vi "Update display current.vi"(8 "error in (no error)":errorcluster, 11 "StageSPIM in":refnum<class "StageSPIM.lvclass">) -> (0 "error out":errorcluster, 3 "StageSPIM out":refnum<class "StageSPIM.lvclass">)   [LabVIEW 2012, in "StageSPIM.lvclass"]
uses:
  StageSPIM.lvclass
  StageSPIM.lvclass/StageSPIM.ctl
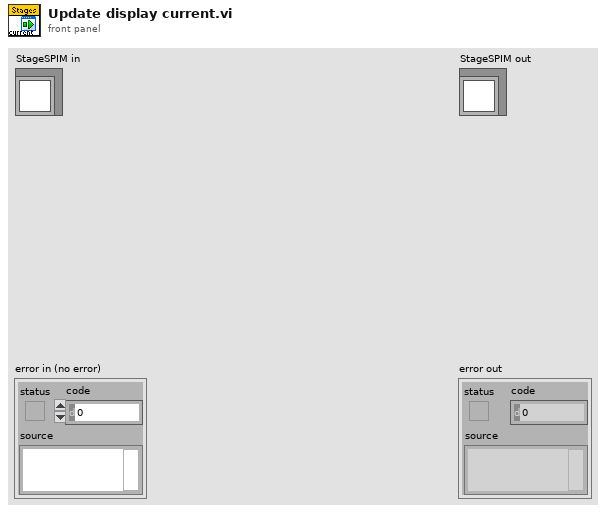
[diagram p1: front panel]
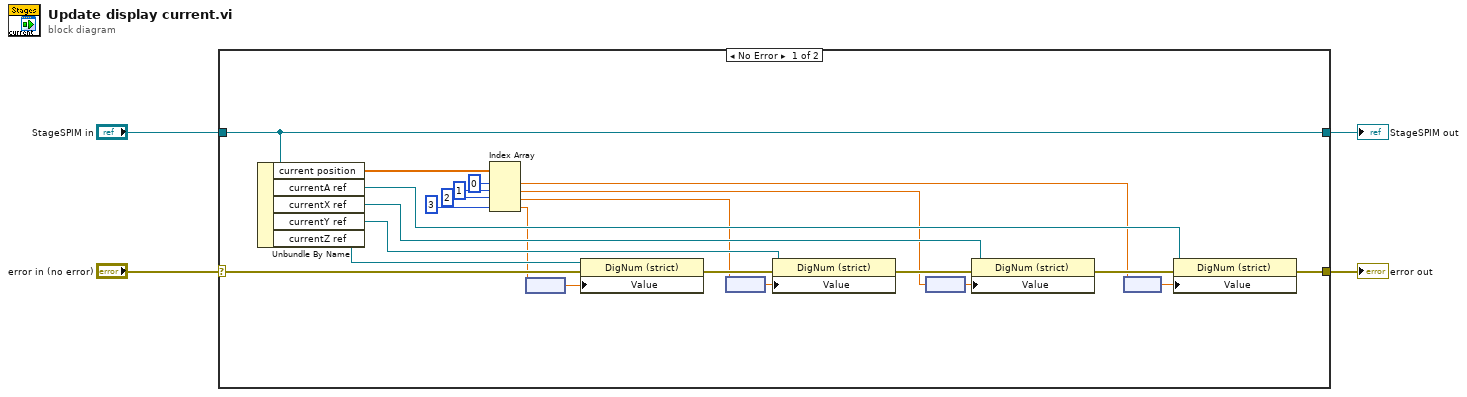
[diagram p0: block diagram]
diagram:
  n1 = case shown="No Error" "error in (no error)" {
    selector: "error in (no error)" -> [w21 w29]
    tunnel: [w13 w29] -> w3
    tunnel: [w27 w28] -> w1
    tunnel: "StageSPIM in" -> [w27 w28]
    frame No Error {
      n2 = Unbundle By Name(w27) -> ("current position"=w26:dbl[], "currentA ref"=w17:refnum<vi>, "currentX ref"=w18:refnum<vi>, "currentY ref"=w19:refnum<vi>, "currentZ ref"=w20:refnum<vi>)
      n3 = Index Array(array=w26, index #1=0 ("index"), index #2=1 ("index"), index #3=2 ("index"), index #4=3 ("index")) -> (element #1=w5:dbl, element #2=w7:dbl, element #3=w9:dbl, element #4=w11:dbl)
      n4 = node(w11) -> (w12:dbl[unit])
      n5 = property class="DigNum (strict)"(reference=w20, error in=w21, "Value"=w12) -> (error out=w16:errorcluster)  [unwired: 1 out]
      n6 = node(w9) -> (w10:dbl[unit])
      n7 = property class="DigNum (strict)"(reference=w19, error in=w16, "Value"=w10) -> (error out=w15:errorcluster)  [unwired: 1 out]
      n8 = node(w7) -> (w8:dbl[unit])
      n9 = property class="DigNum (strict)"(reference=w18, error in=w15, "Value"=w8) -> (error out=w14:errorcluster)  [unwired: 1 out]
      n10 = node(w5) -> (w6:dbl[unit])
      n11 = property class="DigNum (strict)"(reference=w17, error in=w14, "Value"=w6) -> (error out=w13:errorcluster)  [unwired: 1 out]
    }
    frame Error {
    }
  }
  "error out" <- w3
  "StageSPIM out" <- w1
